vi "Self Queue Alias.vi"(11 "Base Queue jettl in":refnum<class "Base Queue jettl.lvclass">) -> (2 "Self Queue Alias":string)   [LabVIEW 2021, in "jettl.lvlib" / "Base Queue jettl.lvlib" / "Base Queue jettl.lvclass"]
uses:
  Base Queue jettl.lvclass
  Base Queue jettl.lvclass/Base Queue jettl.ctl
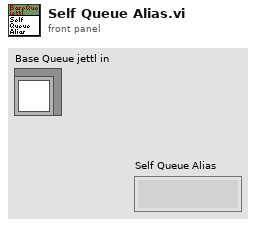
[diagram p1: front panel]
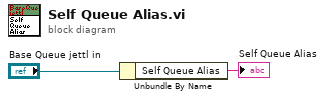
[diagram p0: block diagram]
diagram:
  n1 = Unbundle By Name("Base Queue jettl in") -> ("Self Queue Alias"=→"Self Queue Alias":string)
